vi "题目五.vi"() -> ()   [LabVIEW 2017]
panel:
  in  "停止":bool
  out "显示":T1 {"油量" scale=0.0..100.0; "速度" scale=0.0..300.0; "转速" scale=0.0..8000.0}
  in  "a":dbl
  in  "控制":T2 {"档位" scale=0.0..10.0; "油门" scale=0.0..10.0}
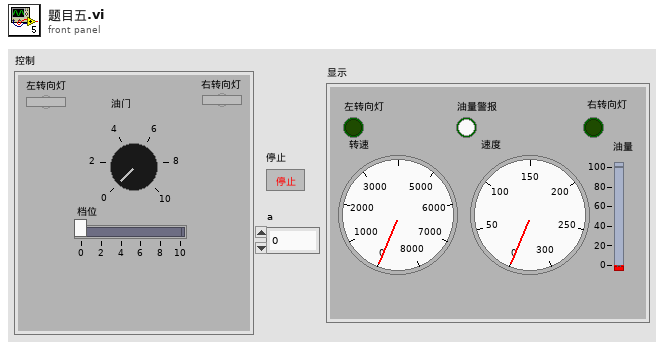
[diagram p1: front panel]
types:
  T1 = cluster{"转速":dbl, "左转向灯":bool, " 右转向灯":bool, "速度":dbl, "油量警报":bool, "油量":dbl}
  T2 = cluster{"油门":dbl, "左转向灯":bool, "右转向灯":bool, "档位":dbl}
  T3 = cluster{dbl, "左转向灯":bool, "右转向灯":bool, dbl, "Blinking":bool, "z":dbl}
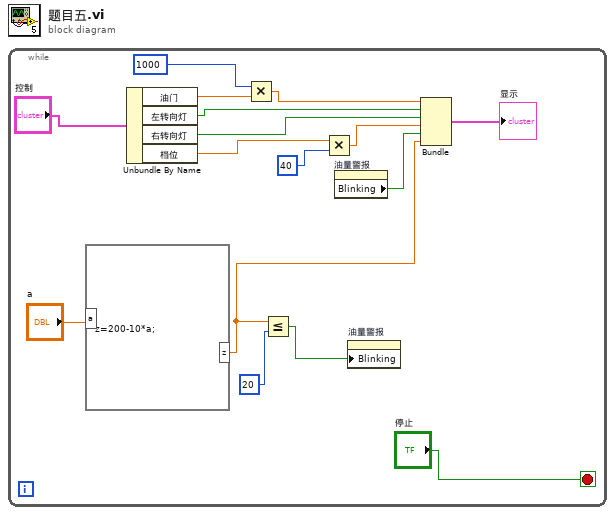
[diagram p0: block diagram]
diagram:
  n1 = while {
    stop <- "停止" stop-if-true
    n2 = formula code="z=200-10*a;"("a"="a") -> ("z"=w3:dbl)
    n3 = Unbundle By Name("控制") -> ("油门"=w11:dbl, "左转向灯"=w9:bool, "右转向灯"=w8:bool, "档位"=w6:dbl)
    n4 = Multiply(x=1000, y=w11) -> (x*y=w10:dbl)
    n5 = Less Or Equal?(x=w3, y=20) -> (x <= y?=w13:bool)
    n6 = Multiply(x=w6, y=40) -> (x*y=w5:dbl)
    n7 = property on="油量警报" class="Bool (严格)"() -> ("Blinking"=w4:bool)  [unwired: 2 in, 2 out]
    n8 = property on="油量警报" class="Bool (严格)"("Blinking"=w13) -> ()  [unwired: 2 in, 2 out]
    n9 = Bundle(w10, "左转向灯"=w9, "右转向灯"=w8, w5, "Blinking"=w4, "z"=w3) -> (→"显示":T3)  [unwired: 1 in]
  }
